vi "Destroy EditPanel.vi"(8 "error in (no error)":errorcluster, 11 "EditPanel in":refnum<class "EditPanel API.lvclass">) -> (0 "error out":errorcluster, 3 "EditPanel out":refnum<class "EditPanel API.lvclass">)   [LabVIEW 2015, in "EditPanel API.lvlib" / "EditPanel API.lvclass"]
uses:
  EditPanel API.lvclass
  EditPanel API.lvclass/EditPanel API.ctl
  Console Reply/Console Reply/Console Reply.lvclass/Console Reply.ctl
  <vilib>/ActorFramework/Stop Msg/Stop Msg.lvclass/Stop Msg.ctl
  <vilib>/ActorFramework/Message Enqueuer/Message Enqueuer.lvclass/Message Enqueuer.ctl
  <vilib>/ActorFramework/Message Enqueuer/Enqueue Critical.vi
  <vilib>/ActorFramework/Message Priority Queue/Priority Enqueue.vi
  <vilib>/ActorFramework/Message Enqueuer/Message Enqueuer.lvclass
  <vilib>/ActorFramework/Stop Msg/Stop Msg.lvclass
  Console Reply/Console Reply/Console Reply.lvclass
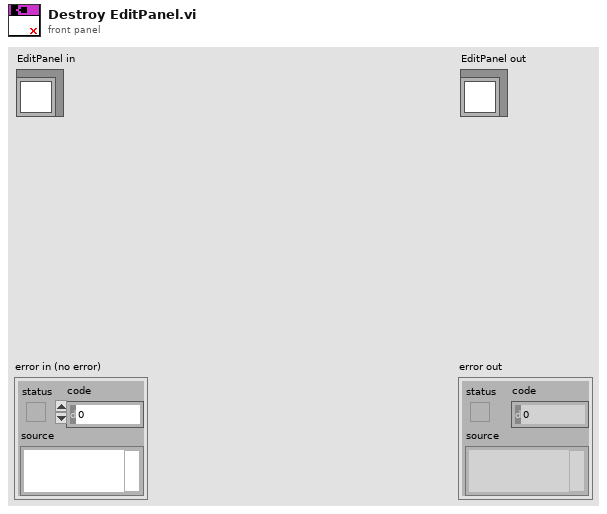
[diagram p1: front panel]
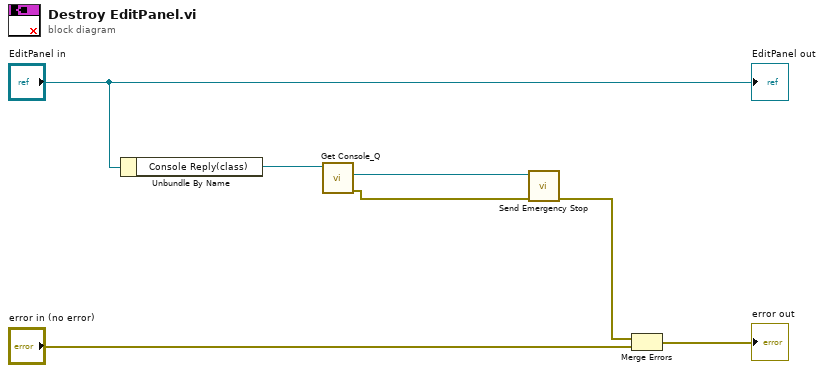
[diagram p0: block diagram]
diagram:
  n1 = Unbundle By Name("EditPanel in") -> ("Console Reply(class)"=w2:refnum<class "Console Reply.lvclass">)
  n2 = call "Get Console_Q.vi"("Console Reply.lvclass"=w2) -> ("error out"=w5:errorcluster, "Console Q"=w6:refnum<class "Message Enqueuer.lvclass">)  [unwired: 8 in, 1 out]
  n3 = call <vilib>:"Send Emergency Stop.vi"("error in (no error)"=w5, "Message Enqueuer"=w6) -> ("error out"=w4:errorcluster)  [unwired: 9 in]
  n4 = Merge Errors(w4, "error in (no error)") -> (→"error out":errorcluster)
  "EditPanel out" <- "EditPanel in"
